vi "Lock Control in The BottomRight.vi"(6 "offset":cluster{"x":i32, "y":i32}, 8 "error in (no error)":errorcluster, 11 "TabControl in":refnum<vi>) -> (0 "error out":errorcluster)   [LabVIEW 2017]
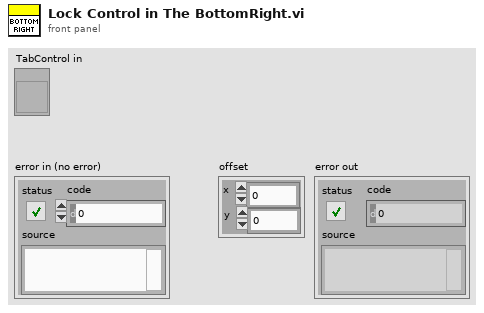
[diagram p1: front panel]
types:
  T1 = typedef "LVBoundsTypeDef.ctl" = cluster{"Width":u32, "Height":u32}
  T2 = typedef "LVPositionTypeDef.ctl" = cluster{"Left":i32, "Top":i32}
  T3 = cluster{"left":i16, "top":i16, "right":i16, "bottom":i16}
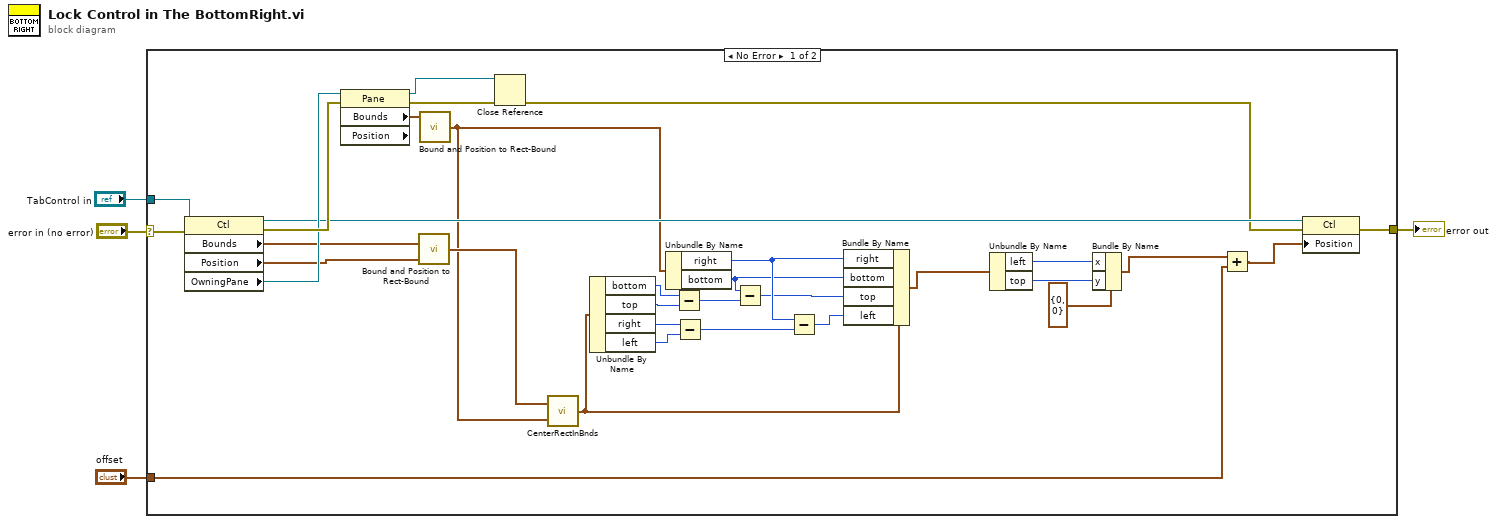
[diagram p0: block diagram]
diagram:
  n1 = case shown="No Error" "error in (no error)" {
    selector: "error in (no error)" -> [w25 w37]
    tunnel: "TabControl in" -> [w27 _]
    tunnel: [w26 w37] -> w3
    tunnel: "offset" -> [w22 _]
    frame No Error {
      n2 = property on="Property Node" class="Ctl"(reference=w27, error in=w25) -> (reference out=w33:refnum<vi>, error out=w35:errorcluster, "Bounds"=w28:T1, "Position"=w29:T2, "OwningPane"=w34:refnum<vi>)
      n3 = property on="Property Node" class="Pane" props=["Bounds", "Position"](reference=w34, error in=w35) -> (reference out=w19:refnum<vi>, error out=w36:errorcluster, "Bounds"=w30:T1)  [unwired: 1 out]
      n4 = call "Bound and Position to Rect-Bound.vi"("Position"=w29, "Bounds"=w28) -> ("Rect Bound"=w32:T3)  [unwired: 3 in]
      n5 = call "Bound and Position to Rect-Bound.vi"("Bounds"=w30) -> ("Rect Bound"=w31:T3)  [unwired: 4 in]
      n6 = Close Reference(reference=w19, error in (no error)=w36) -> (error out=w20:errorcluster)
      n7 = call <vilib>:"CenterRectInBnds.vi"("bounds"=w31, "rect"=w32) -> ("centered rect"=w11:T3)
      n8 = Unbundle By Name(w11) -> ("bottom"=w8:i16, "top"=w9:i16, "right"=w14:i16, "left"=w15:i16)
      n9 = Unbundle By Name(w31) -> ("right"=w16:i16, "bottom"=w13:i16)
      n10 = Subtract(x=w8, y=w9) -> (x-y=w10:i16)
      n11 = Subtract(x=w14, y=w15) -> (x-y=w17:i16)
      n12 = Subtract(x=w13, y=w10) -> (x-y=w12:i16)
      n13 = Subtract(x=w16, y=w17) -> (x-y=w18:i16)
      n14 = Bundle By Name(cluster=w11, "right"=w16, "bottom"=w13, "top"=w12, "left"=w18) -> (w24:T3)
      n15 = Unbundle By Name(w24) -> ("left"=w6:i16, "top"=w7:i16)
      n16 = Bundle By Name(cluster=cluster{"x":i32, "y":i32} {"x"=0, "y"=0} ("Point"), "x"=w6, "y"=w7) -> (w23:cluster{"x":i32, "y":i32})
      n17 = Add(x=w23, y=w22) -> (x+y=w21:cluster{"x":i32, "y":i32})
      n18 = property on="Property Node" class="Ctl"(reference=w33, error in=w20, "Position"=w21) -> (error out=w26:errorcluster)  [unwired: 1 out]
    }
    frame Error {
    }
  }
  "error out" <- w3
